vi "log_viewer.vi"() -> ()   [LabVIEW 2012]
uses:
  testing/log_event.ctl
panel:
  out "Selected":u32
  out "Event count":i32
  in  "stop":bool
  out "Event log":T1[](array[typedef]) {"Timestamp" format="%<%.3X>T"}
  out "File exists":bool
  in  "Input file":path
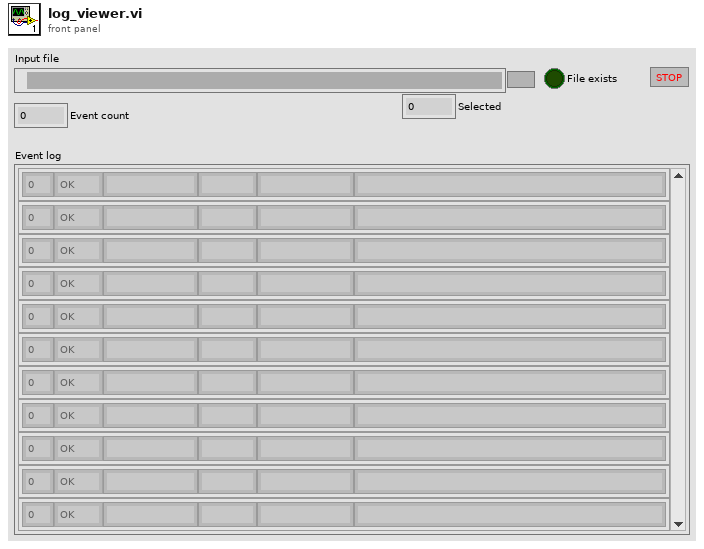
[diagram p1: front panel]
types:
  T1 = typedef "log_event.ctl" = cluster{"Facility ID":i32, "Severity":enum16{"OK", "Debug", "Warn", "Error"}, "Timestamp":timestamp, "Facility":string, "State":string, "Message":string}
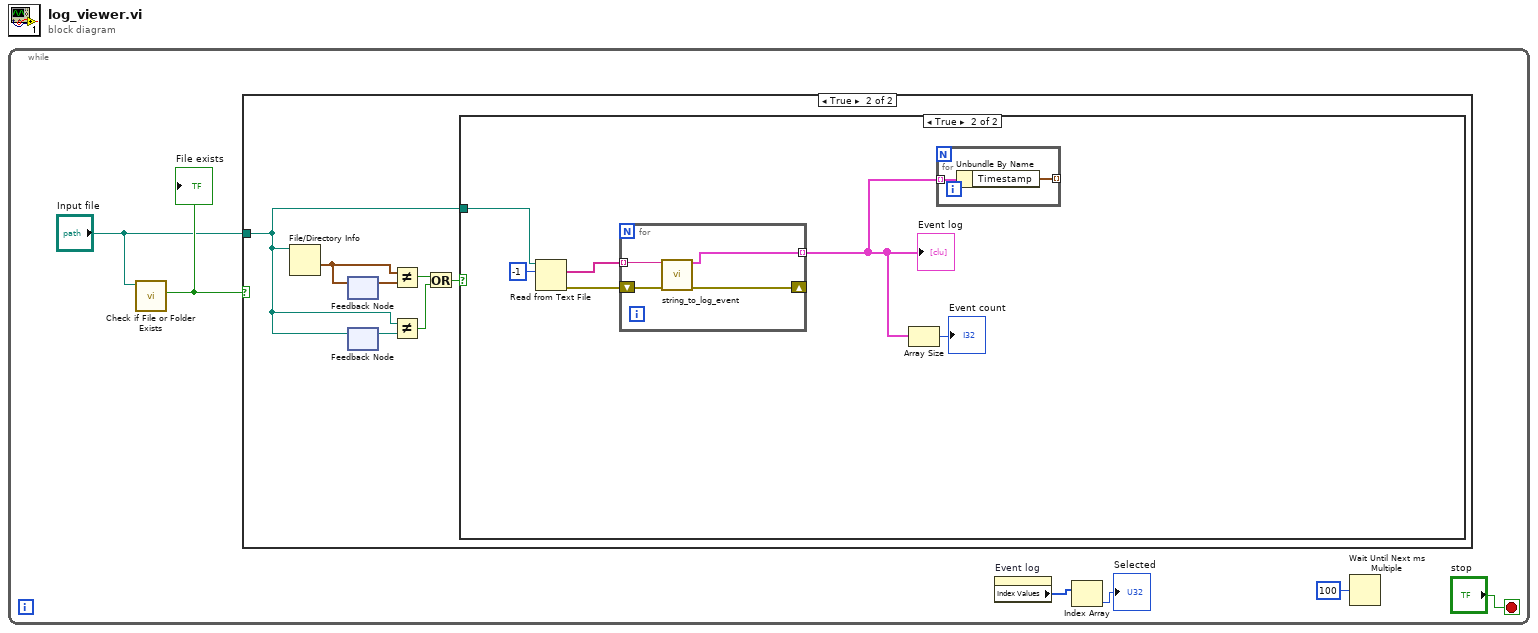
[diagram p0: block diagram]
diagram:
  n1 = while {
    stop <- "stop" stop-if-true
    n2 = call <vilib>:"Check if File or Folder Exists.vi"("path"="Input file") -> ("file or folder exists?"=w6:bool)  [unwired: 8 in, 2 out]
    "File exists" <- w6
    n3 = case shown="True" w6 {
      tunnel: "Input file" -> [_ w10]
      frame False {
      }
      frame True {
        n4 = File/Directory Info(path=w10) -> (last mod=w11:timestamp)  [unwired: 1 in, 6 out]
        n5 = feedback #1() -> (w12:timestamp)  [unwired: 1 in]
        n6 = feedback-in #1(w11) -> ()
        n7 = feedback #2() -> (w13:path)  [unwired: 1 in]
        n8 = feedback-in #2(w10) -> ()
        n9 = Not Equal?(x=w11, y=w12) -> (x != y?=w9:bool)
        n10 = Not Equal?(x=w10, y=w13) -> (x != y?=w8:bool)
        n11 = Or(x=w9, y=w8) -> (x .or. y?=w7:bool)
        n12 = case shown="True" w7 {
          tunnel: w10 -> [_ w18]
          frame False {
          }
          frame True {
            n13 = Read from Text File(file (use dialog)=w18, count=-1) -> (text=w17:string[], error out=w16:errorcluster)  [unwired: 2 in, 2 out]
            n14 = for {
              tunnel: w17 -> [w25] mode=indexing
              shift-right: [w22] -> _
              shift-left: w16 -> [w24]
              tunnel: [w23] -> w14 mode=indexing
              n15 = call "string_to_log_event.vi"("String"=w25, "error in"=w24) -> ("Log event"=w23:T1, "error out"=w22:errorcluster)  [unwired: 12 in]
            }
            "Event log" <- w14
            n16 = Array Size(array=w14) -> (size(s)=→"Event count":i32)
            n17 = for {
              tunnel: w14 -> [w21] mode=indexing
              tunnel: [w20] -> _ mode=indexing
              n18 = Unbundle By Name(w21) -> ("Timestamp"=w20:timestamp)
            }
          }
        }
      }
    }
    n19 = property on="Event log" class="Arr (strict)"() -> ("Index Values"=w2:u32[])  [unwired: 2 in, 2 out]
    n20 = Index Array(array=w2) -> (element=→"Selected":u32)  [unwired: 1 in]
    n21 = Wait Until Next ms Multiple(millisecond multiple=u32 100) -> ()  [unwired: 1 out]
  }
